vi "AudioTest.Check if Mic and Speaker Operate.vi"() -> ()   [LabVIEW 2018]
uses:
  Functional Test/TypeDefs/FunctTest.Test Item with 2D Image for Instructions, Pass is Indicator Only.ctl
  Functional Test/TypeDefs/FunctTest.Result State.ctl
  Common/Instruments/Audio/Audio Play Record/Audio.Play Signal Setup.ctl
  Common/Instruments/Audio/Audio Play Record/Audio.Record Signal Setup.ctl
  <vilib>/KATE/Queues/Queue Utils.lvlib
panel:
  out "CL Args":string[](array[string])
  out "Output file":path
  out "error out":errorcluster
  out "Running":bool
  in  "Run All Audio Tests":bool
  in  "Run Audio Right Test":bool
  in  "Run Audio Left Test":bool
  in  "Run Audio Mic Test":bool
  out "Test Run Time(s)":dbl format="%.3f"
  out "Left Speaker Spectrum":T1(graph)
  out "Left Test Result":T2
  out "Left Rec Tones (Hz)":dbl[](array[numeric])
  out "Right Rec Tones (Hz)":dbl[](array[numeric])
  out "Right Speaker Spectrum":T1(graph)
  out "Right Test Result":T2
  out "Mic Rec Tones (Hz)":dbl[](array[numeric])
  out "Microphone Spectrum":T1(graph)
  out "Mic Test Result":T2
  in  "Tol%":dbl=3.0 caption="Tone Tolerance(+/-%)"
  in  "RtSetup":T3={"Play Device"="Utah", "Play Volume"=90.0, "DTMF Channel"=7, "Rec Device"="Jabra"} caption="Right Speaker Test Setup"
  in  "LftSetup":T3={"Play Device"="Utah", "Play Volume"=90.0, "DTMF Channel"=4, "Rec Device"="Jabra"} caption="Left Speaker Test Setup"
  in  "MicSetup":T3={"Play Device"="Jabra", "Play Volume"=60.0, "DTMF Channel"=1, "Rec Device"="Valve"} caption="Microphone Test Setup"
  in  "ToneThr":dbl=0.0005 caption="Tone Threshold"
  in  "Sample Rate":dbl=44100.0
  in  "ToneDur":dbl=0.35 caption="Tone Duration(s)"
  out "Audio Test":T4
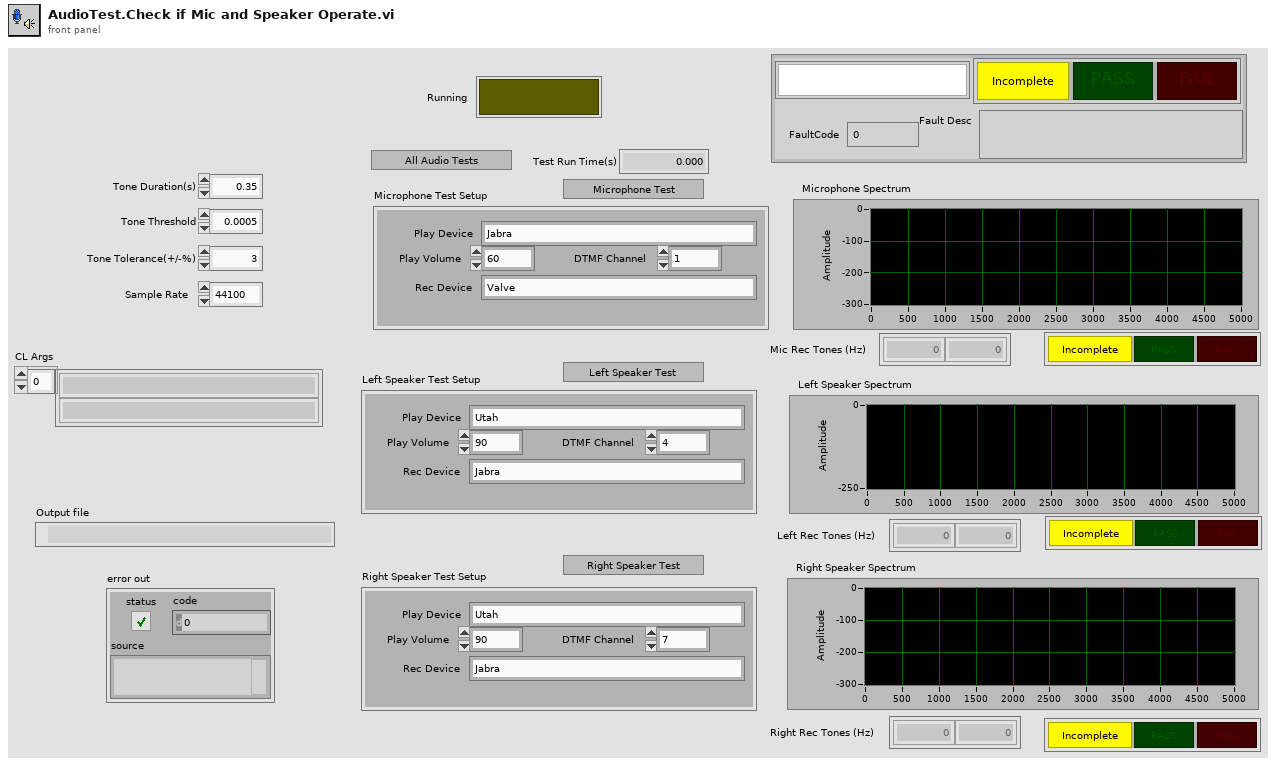
[diagram p1: front panel]
types:
  T1 = cluster{"f0":dbl, "df":dbl, "dB Spectrum (Hann)":dbl[]}
  T2 = typedef "FunctTest.Result State.ctl" = enum32{"NoTest", "PASS", "FAIL"}
  T3 = cluster{"Play Device":string, "Play Volume":dbl, "DTMF Channel":i32, "Rec Device":string}
  T4 = typedef "FunctTest.Test Item with 2D Image for Instructions, Pass is Indicator Only.ctl" = cluster{"Name":picture, "Result":T2, "FaultCode":i32, "Fault Desc":string, "Disabled":bool}
  T5 = enum32{"invalid app kind", "Development System", "Run Time System", "Student Edition", "Embedded LabVIEW", "Evaluation", "Custom"}
  T6 = enum32{"Invalid", "Standard", "Closed", "Hidden", "Minimized", "Maximized"}
  T7 = typedef "Audio.Record Signal Setup.ctl" = cluster{"Device":string, "Left En":bool, "Right En":bool, "PrePlaySec":dbl, "PostPlaySec":dbl}
  T8 = typedef "Audio.Play Signal Setup.ctl" = cluster{"Device":string, "Left En":bool, "Right En":bool, "Volume(%)":dbl, "Amplitude":dbl}
  T9 = cluster{"ToneDur":dbl, "Sample Rate":dbl, "ToneThr":dbl, "Tol%":dbl, "MicSetup":cluster{"Play Device":string, "Play Volume":dbl, "DTMF Channel":i32, "Rec Device":string}, "RtSetup":cluster{"Play Device":string, "Play Volume":dbl, "DTMF Channel":i32, "Rec Device":string}, "LftSetup":cluster{"Play Device":string, "Play Volume":dbl, "DTMF Channel":i32, "Rec Device":string}, "Start":dbl, "CLI":string[], "Out Dir":path, "Faults":errorcluster[]}
  T10 = cluster{"frequency":dbl, "amplitude":dbl, "phase":dbl}[]
  T11 = cluster{"detected frequency":dbl, "detected amplitude":dbl, "detected phase (deg)":dbl}[]
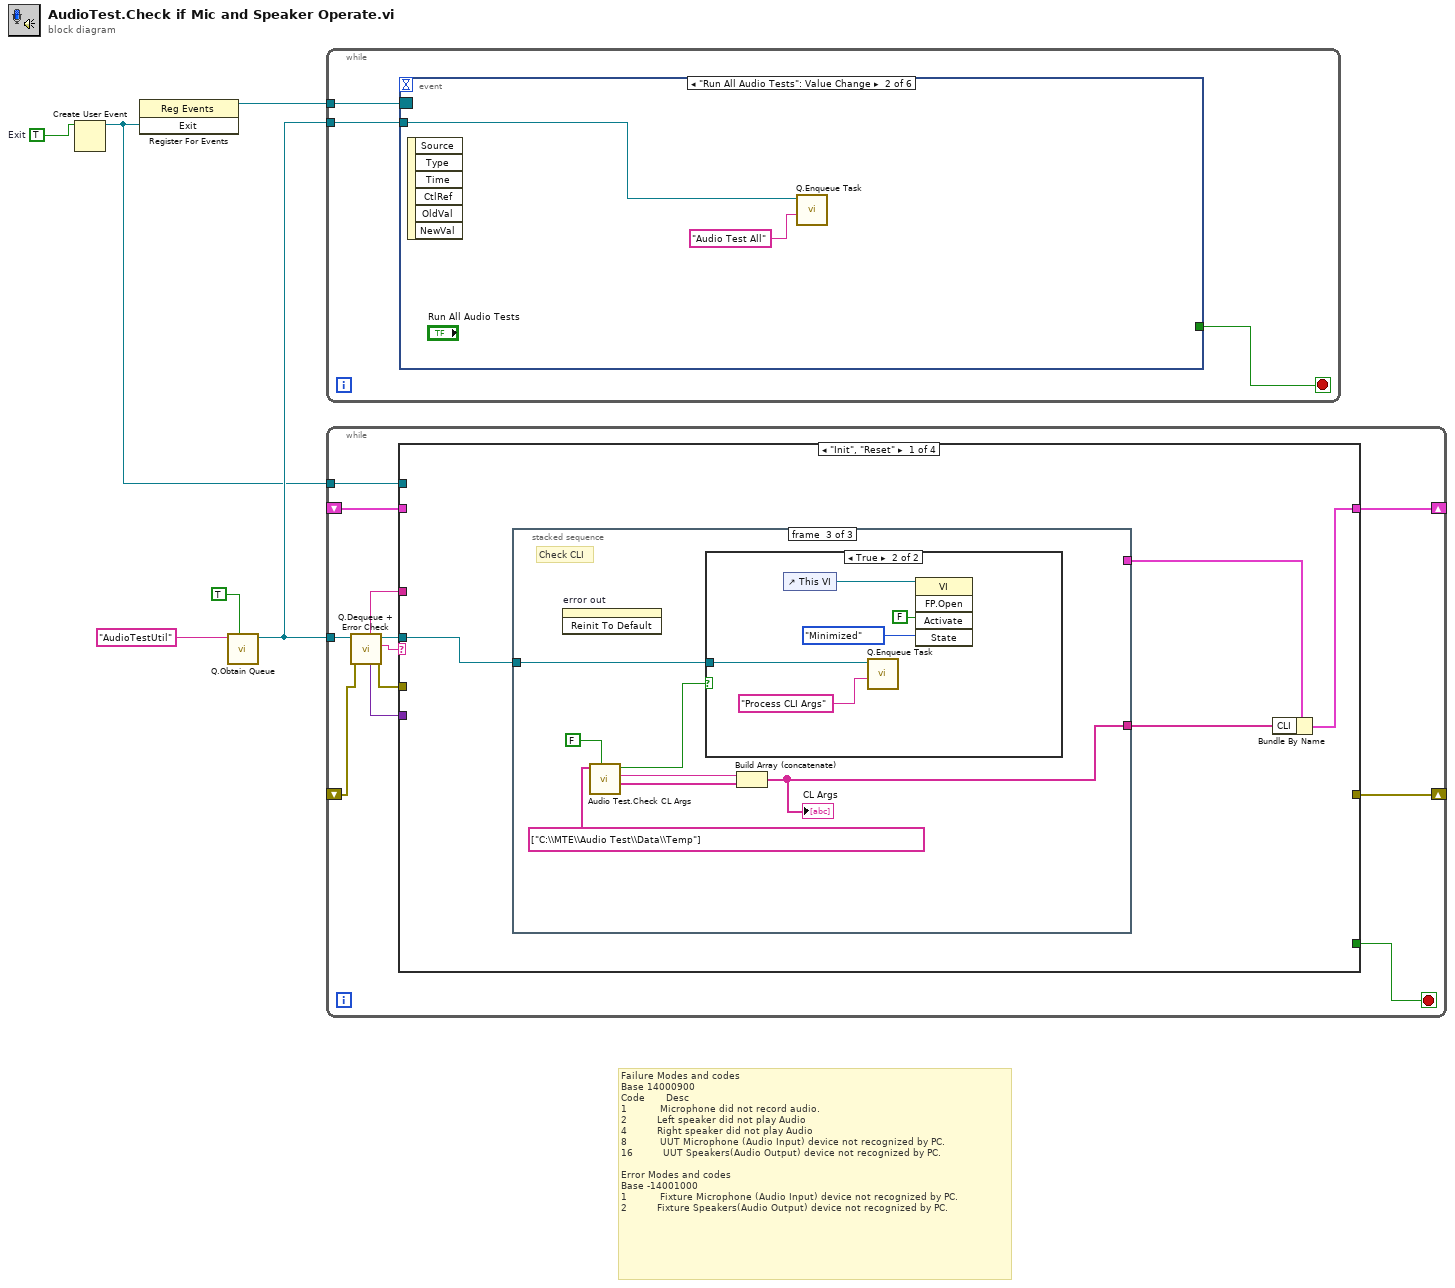
[diagram p0: block diagram]
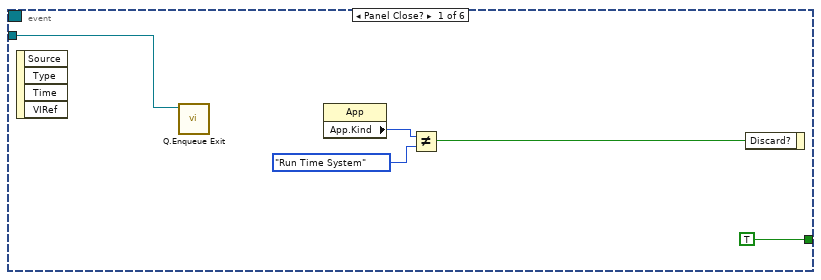
[diagram p2: hidden frame]
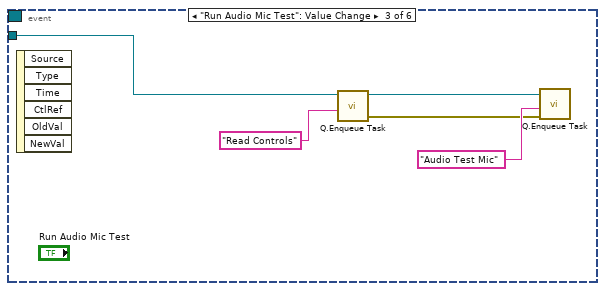
[diagram p3: hidden frame]
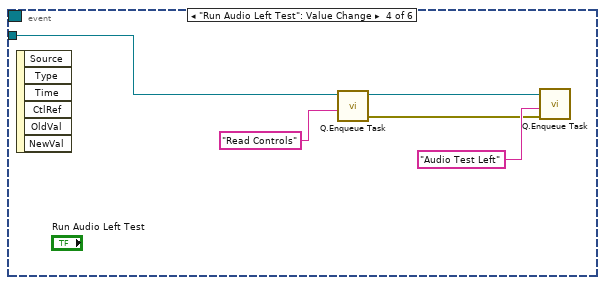
[diagram p4: hidden frame]
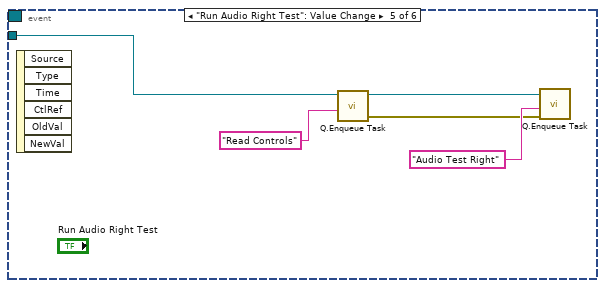
[diagram p5: hidden frame]
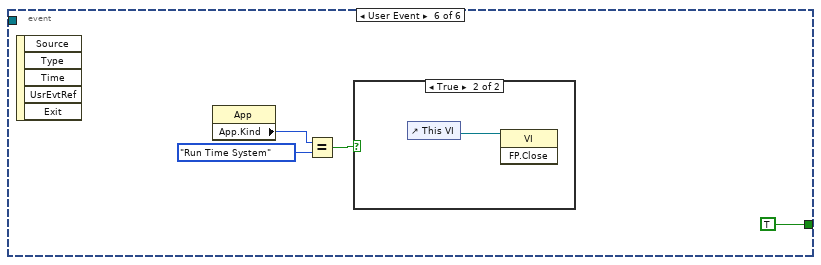
[diagram p6: hidden frame]
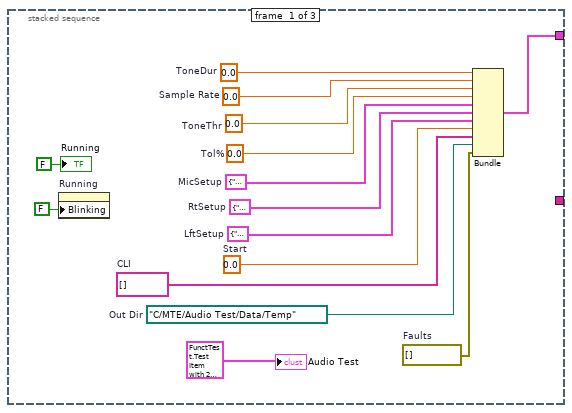
[diagram p8: hidden frame]
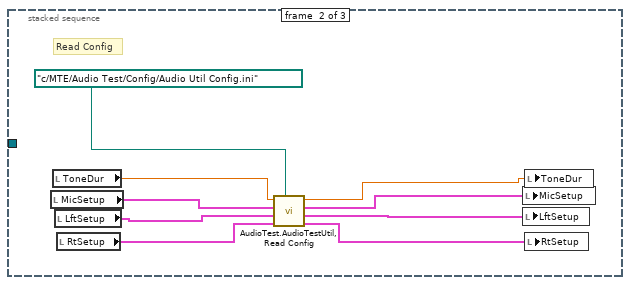
[diagram p9: hidden frame]
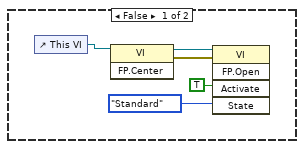
[diagram p10: hidden frame]
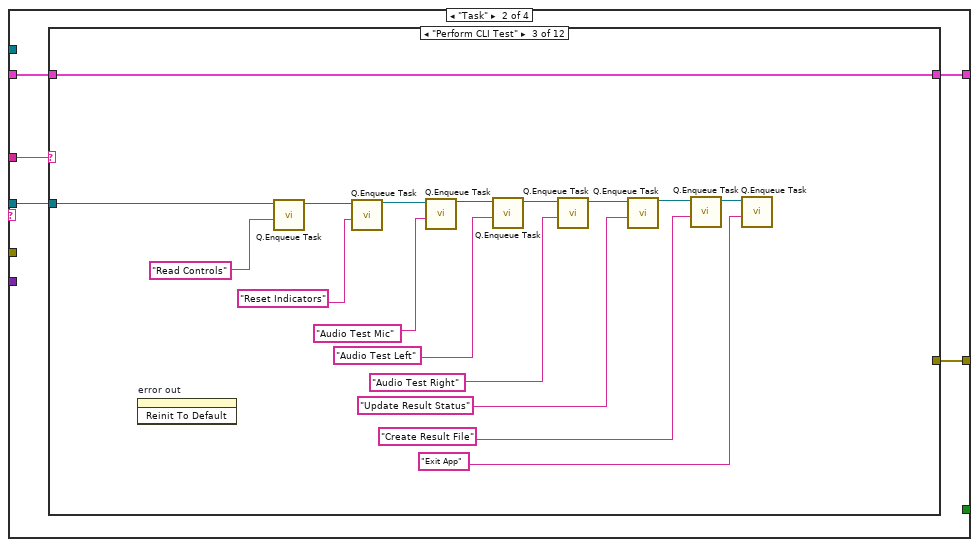
[diagram p11: hidden frame]
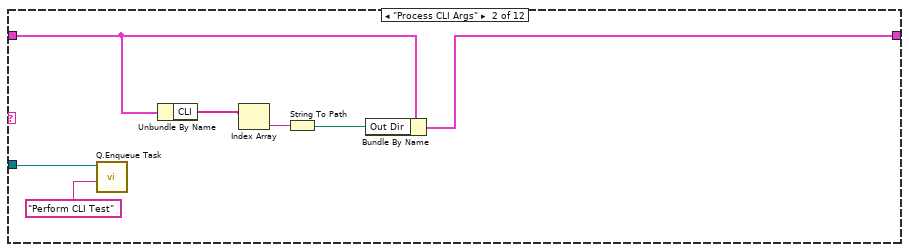
[diagram p13: hidden frame]
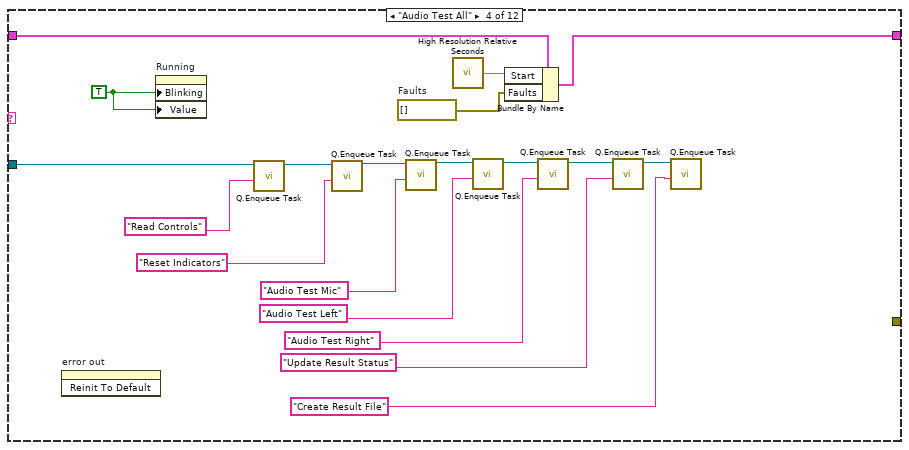
[diagram p14: hidden frame]
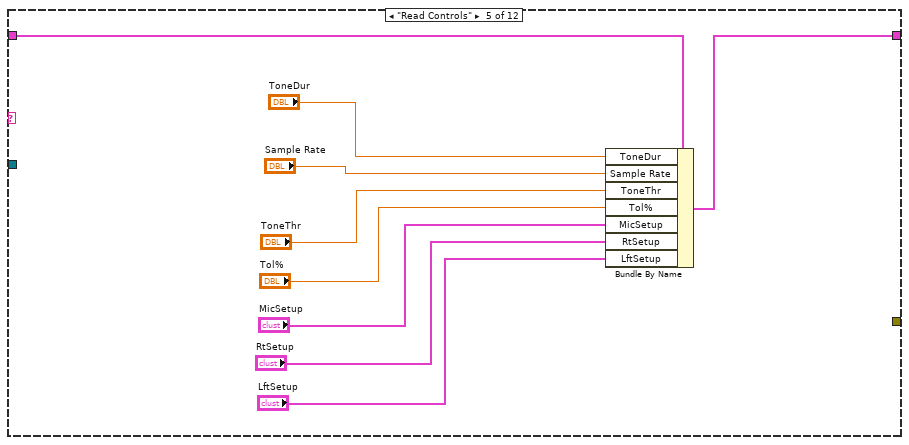
[diagram p15: hidden frame]
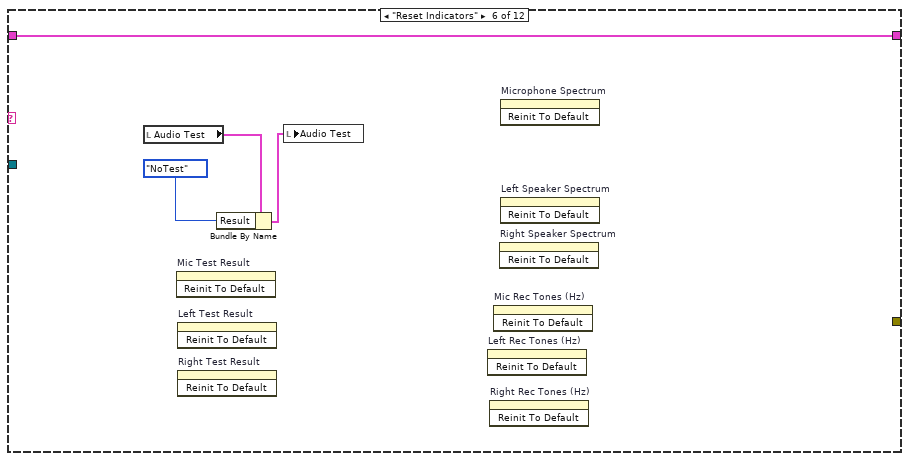
[diagram p16: hidden frame]
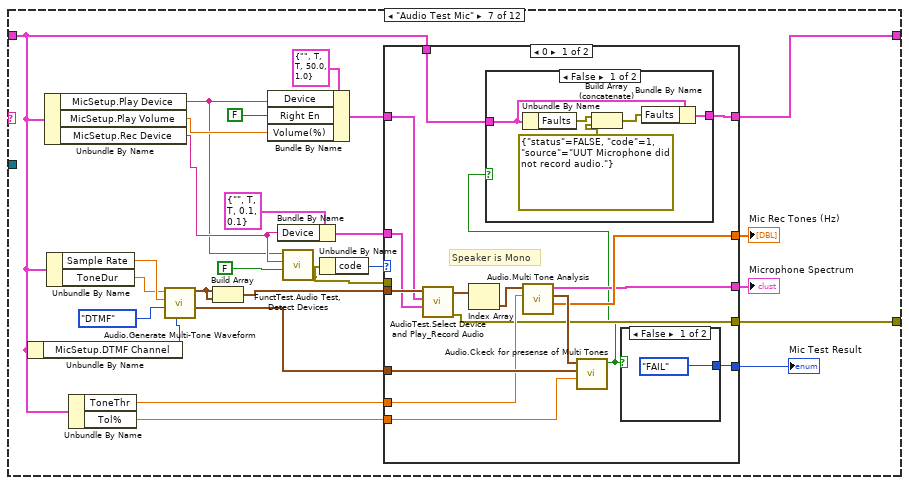
[diagram p17: hidden frame]
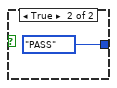
[diagram p19: hidden frame]
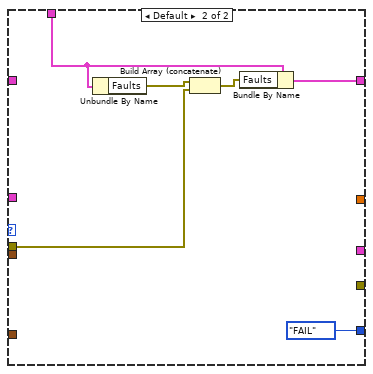
[diagram p20: hidden frame]
diagram:
  w2 = TRUE  # Exit
  # "Failure Modes and codes\nBase 14000900\nCode       Desc\n1           Microphone did not record audio.\n2          Left speaker did not play Audio\n4          Right speaker did not play Audio\n8           UUT Microphone (Audio Input) device not recognized by PC.\n16          UUT Speakers(Audio Output) device not recognized by PC.\n\nError Modes and codes\nBase -14001000\n1           Fixture Microphone (Audio Input) device not recognized by PC.\n2          Fixture Speakers(Audio Output) device not recognized by PC."
  n1 = Create User Event(user event datatype=w2) -> (user event=w1:refnum<user-event>)  [unwired: 1 in, 1 out]
  n2 = register-events(w1) -> (reference out=w3:refnum<event-registration>)  [unwired: 2 in, 1 out]
  n3 = call <vilib>:"Q.Obtain Queue.vi"("Enqueue Init"=TRUE, "Q Name"="AudioTestUtil") -> ("Q Out"=w4:refnum<queue>)  [unwired: 7 in, 2 out]
  n4 = while {
    tunnel: w4 -> [w8]
    tunnel: w3 -> [w7]
    stop <- w9 stop-if-true
    n5 = event shown="[1] \"Run All Audio Tests\": Value Change" {
      selector: w7 -> [_ _ _ _ _ _]
      dyn-events: _ -> [_ _ _ _ _ _]
      timeout: _ -> [_ _ _ _ _ _]
      tunnel: [TRUE _ _ _ _ TRUE] -> w9
      tunnel: w8 -> [w10 w15 w18 w23 w28 _]
      event Panel Close? {
        n6 = event-data() -> ()  [unwired: 1 in, 4 out]
        n7 = call <vilib>:"Q.Enqueue Exit.vi"("Q In"=w10) -> ()  [unwired: 9 in, 2 out]
        n8 = property class="App"() -> ("App.Kind"=w14:T5)  [unwired: 2 in, 2 out]
        n9 = Not Equal?(x=w14, y=T5."Run Time System") -> (x != y?=w12:bool)
        n10 = event-data("Discard?"=w12) -> ()  [unwired: 1 in, 1 out]
      }
      event "Run All Audio Tests": Value Change {
        n11 = event-data() -> ()  [unwired: 1 in, 6 out]
        n12 = call <vilib>:"Q.Enqueue Task.vi"("Task Name"="Audio Test All", "Q In"=w15) -> ()  [unwired: 8 in, 2 out]
      }
      event "Run Audio Mic Test": Value Change {
        n13 = event-data() -> ()  [unwired: 1 in, 6 out]
        n14 = call <vilib>:"Q.Enqueue Task.vi"("Task Name"="Read Controls", "Q In"=w18) -> ("error out"=w19:errorcluster, "Q Out"=w17:refnum<queue>)  [unwired: 8 in]
        n15 = call <vilib>:"Q.Enqueue Task.vi"("Error In"=w19, "Task Name"="Audio Test Mic", "Q In"=w17) -> ()  [unwired: 7 in, 2 out]
      }
      event "Run Audio Left Test": Value Change {
        n16 = event-data() -> ()  [unwired: 1 in, 6 out]
        n17 = call <vilib>:"Q.Enqueue Task.vi"("Task Name"="Read Controls", "Q In"=w23) -> ("error out"=w24:errorcluster, "Q Out"=w22:refnum<queue>)  [unwired: 8 in]
        n18 = call <vilib>:"Q.Enqueue Task.vi"("Error In"=w24, "Task Name"="Audio Test Left", "Q In"=w22) -> ()  [unwired: 7 in, 2 out]
      }
      event "Run Audio Right Test": Value Change {
        n19 = event-data() -> ()  [unwired: 1 in, 6 out]
        n20 = call <vilib>:"Q.Enqueue Task.vi"("Task Name"="Read Controls", "Q In"=w28) -> ("error out"=w29:errorcluster, "Q Out"=w27:refnum<queue>)  [unwired: 8 in]
        n21 = call <vilib>:"Q.Enqueue Task.vi"("Error In"=w29, "Task Name"="Audio Test Right", "Q In"=w27) -> ()  [unwired: 7 in, 2 out]
      }
      event User Event {
        n22 = event-data() -> ()  [unwired: 1 in, 5 out]
        n23 = property class="App"() -> ("App.Kind"=w34:T5)  [unwired: 2 in, 2 out]
        n24 = Equal?(x=w34, y=T5."Run Time System") -> (x = y?=w32:bool)
        n25 = case shown="True" w32 {
          frame False {
          }
          frame True {
            n26 = control-ref of="This VI"() -> (w36:refnum<vi>)
            n27 = invoke class="VI" method="FP.Close"(reference=w36) -> ()  [unwired: 2 in, 3 out]
          }
        }
      }
    }
  }
  n28 = while {
    tunnel: w4 -> [w45]
    shift-right: [w43] -> _
    shift-left: _ -> [w44]
    shift-right: [w41] -> _
    shift-left: _ -> [w40]
    tunnel: w1 -> [w38]
    stop <- w42 stop-if-true
    n29 = call <vilib>:"Q.Dequeue + Error Check.vi"("Error In"=w40, "Q In"=w45) -> ("error out"=w39:errorcluster, "Cmd"=w48:string, "Q Out"=w47:refnum<queue>, "Data1"=w37:variant, "Sub"=w46:string)  [unwired: 4 in, 1 out]
    n30 = case shown="\"Init\", \"Reset\"" w48 {
      tunnel: w47 -> [w52 w94 _ _]
      tunnel: w46 -> [_ w98 w410 _]
      tunnel: w44 -> [_ w97 w411 w419]
      tunnel: [w50 w96 w411 w419] -> w43
      tunnel: [_ _ _ TRUE] -> w42
      tunnel: [_ w95 _ _] -> w41
      tunnel: w39 -> [_ _ w409 _]
      tunnel: w38 -> [_ _ _ w417]
      tunnel: w37 -> [_ _ w408 _]
      frame "Init", "Reset" {
        n31 = stacked-sequence {
          tunnel: [w60 _ _] -> w51
          tunnel: w52 -> [_ _ w83]
          tunnel: [_ _ w78] -> w49
          frame #0 {
            w53 = errorcluster[] []  # Faults
            w54 = path "C:/MTE/Audio Test/Data/Temp"  # Out Dir
            w55 = string[] []  # CLI
            w59 = 0.0  # Start
            w61 = T3 {"Play Device"="", "Play Volume"=0.0, "DTMF Channel"=0, "Rec Device"=""}  # LftSetup
            w62 = T3 {"Play Device"="", "Play Volume"=0.0, "DTMF Channel"=0, "Rec Device"=""}  # RtSetup
            w63 = T3 {"Play Device"="", "Play Volume"=0.0, "DTMF Channel"=0, "Rec Device"=""}  # MicSetup
            w64 = 0.0  # Tol%
            w65 = 0.0  # ToneThr
            w66 = 0.0  # Sample Rate
            w67 = 0.0  # ToneDur
            n32 = property on="Running" class="Bool (strict)"("Blinking"=FALSE) -> ()  [unwired: 2 in, 2 out]
            n33 = Bundle("ToneDur"=w67, "Sample Rate"=w66, "ToneThr"=w65, "Tol%"=w64, "MicSetup"=w63, "RtSetup"=w62, "LftSetup"=w61, "Start"=w59, "CLI"=w55, "Out Dir"=w54, "Faults"=w53) -> (w60:T9)  [unwired: 1 in]
            "Running" <- FALSE ("Running")
            "Audio Test" <- T4 {"Name"=bytes[74], "Result"=enum."NoTest", "FaultCode"=0, "Fault Desc"="", "Disabled"=TRUE} ("Audio Test")
          }
          frame #1 {
            # "Read Config"
            n34 = local read "MicSetup"() -> (w74:T3)
            n35 = local read "ToneDur"() -> (w76:dbl)
            n36 = local read "LftSetup"() -> (w73:T3)
            n37 = local read "RtSetup"() -> (w72:T3)
            n38 = call "AudioTest.AudioTestUtil, Read Config.vi"("File"=path "c:/MTE/Audio Test/Config/Audio Util Config.ini", "RtSetup"=w72, "LftSetup"=w73, "MicSetup"=w74, "ToneDur"=w76) -> ("RtSetup Out"=w68:T3, "LftSetup Out"=w69:T3, "MicSetup Out"=w70:T3, "ToneDur Out"=w71:dbl)  [unwired: 2 in, 1 out]
            n39 = local write "MicSetup"(w70) -> ()
            n40 = local write "LftSetup"(w69) -> ()
            n41 = local write "ToneDur"(w71) -> ()
            n42 = local write "RtSetup"(w68) -> ()
          }
          frame #2 {
            # "Check CLI"
            n43 = invoke on="error out" class="Clust (strict)" method="Reinit To Default"() -> ()  [unwired: 3 in, 3 out]
            n44 = call "Audio Test.Check CL Args.vi"("Simulate"=FALSE, "Sim CL Args"=string[] ["C:\\MTE\\Audio Test\\Data\\Temp"]) -> ("Args"=w77:string[], "Action"=w81:string, "CmdLine"=w82:bool)  [unwired: 7 in]
            n45 = case shown="True" w82 {
              tunnel: w83 -> [_ w92]
              frame False {
                n46 = control-ref of="This VI"() -> (w86:refnum<vi>)
                n47 = invoke class="VI" method="FP.Center"(reference=w86) -> (reference out=w87:refnum<vi>, error out=w88:errorcluster)  [unwired: 2 in, 1 out]
                n48 = invoke class="VI" method="FP.Open"(reference=w87, error in=w88, "Activate"=TRUE ("Activate?"), "State"=T6."Standard") -> ()  [unwired: 1 in, 5 out]
              }
              frame True {
                n49 = control-ref of="This VI"() -> (w89:refnum<vi>)
                n50 = call <vilib>:"Q.Enqueue Task.vi"("Task Name"="Process CLI Args", "Q In"=w92) -> ()  [unwired: 8 in, 2 out]
                n51 = invoke class="VI" method="FP.Open"(reference=w89, "Activate"=FALSE ("Activate?"), "State"=T6."Minimized") -> ()  [unwired: 2 in, 5 out]
              }
            }
            n52 = Build Array (concatenate)(w81, w77) -> (w78:string[])
            "CL Args" <- w78
          }
        }
        n53 = Bundle By Name(cluster=w51, "CLI"=w49) -> (w50:T9)
      }
      frame "Task" {
        n54 = case shown="\"Perform CLI Test\"" w98 {
          tunnel: w97 -> [w99 w100 w123 w128 w143 w155 w156 w215 w271 w338 w404 w406]
          tunnel: [w99 w101 w123 w129 w144 w155 w157 w213 w268 w338 w404 w406] -> w96
          tunnel: [_ _ _ _ _ _ w172 w228 w283 _ w389 _] -> w95
          tunnel: w94 -> [_ w105 w111 w131 _ _ _ _ _ _ _ w405]
          frame Default {
          }
          frame "Process CLI Args" {
            n55 = call <vilib>:"Q.Enqueue Task.vi"("Task Name"="Perform CLI Test", "Q In"=w105) -> ()  [unwired: 8 in, 2 out]
            n56 = Unbundle By Name(w100) -> ("CLI"=w104:string[])
            n57 = Index Array(array=w104) -> (element=w103:string)  [unwired: 1 in]
            n58 = String To Path(string=w103) -> (path=w102:path)
            n59 = Bundle By Name(cluster=w100, "Out Dir"=w102) -> (w101:T9)
          }
          frame "Perform CLI Test" {
            n60 = invoke on="error out" class="Clust (strict)" method="Reinit To Default"() -> ()  [unwired: 3 in, 3 out]
            n61 = call <vilib>:"Q.Enqueue Task.vi"("Task Name"="Read Controls", "Q In"=w111) -> ("Q Out"=w113:refnum<queue>)  [unwired: 8 in, 1 out]
            n62 = call <vilib>:"Q.Enqueue Task.vi"("Task Name"="Reset Indicators", "Q In"=w113) -> ("Q Out"=w117:refnum<queue>)  [unwired: 8 in, 1 out]
            n63 = call <vilib>:"Q.Enqueue Task.vi"("Task Name"="Audio Test Mic", "Q In"=w117) -> ("Q Out"=w122:refnum<queue>)  [unwired: 8 in, 1 out]
            n64 = call <vilib>:"Q.Enqueue Task.vi"("Task Name"="Audio Test Left", "Q In"=w122) -> ("Q Out"=w121:refnum<queue>)  [unwired: 8 in, 1 out]
            n65 = call <vilib>:"Q.Enqueue Task.vi"("Task Name"="Audio Test Right", "Q In"=w121) -> ("Q Out"=w115:refnum<queue>)  [unwired: 8 in, 1 out]
            n66 = call <vilib>:"Q.Enqueue Task.vi"("Task Name"="Update Result Status", "Q In"=w115) -> ("Q Out"=w110:refnum<queue>)  [unwired: 8 in, 1 out]
            n67 = call <vilib>:"Q.Enqueue Task.vi"("Task Name"="Create Result File", "Q In"=w110) -> ("Q Out"=w108:refnum<queue>)  [unwired: 8 in, 1 out]
            n68 = call <vilib>:"Q.Enqueue Task.vi"("Task Name"="Exit App", "Q In"=w108) -> ()  [unwired: 8 in, 2 out]
          }
          frame "Audio Test All" {
            w124 = errorcluster[] []  # Faults
            w133 = TRUE ("Blinking")
            n69 = invoke on="error out" class="Clust (strict)" method="Reinit To Default"() -> ()  [unwired: 3 in, 3 out]
            n70 = property on="Running" class="Bool (strict)"("Blinking"=w133, "Value"=w133) -> ()  [unwired: 2 in, 2 out]
            n71 = call <vilib>:"Q.Enqueue Task.vi"("Task Name"="Read Controls", "Q In"=w131) -> ("Q Out"=w132:refnum<queue>)  [unwired: 8 in, 1 out]
            n72 = call <vilib>:"Q.Enqueue Task.vi"("Task Name"="Reset Indicators", "Q In"=w132) -> ("Q Out"=w137:refnum<queue>)  [unwired: 8 in, 1 out]
            n73 = call <vilib>:"Q.Enqueue Task.vi"("Task Name"="Audio Test Mic", "Q In"=w137) -> ("Q Out"=w142:refnum<queue>)  [unwired: 8 in, 1 out]
            n74 = call <vilib>:"High Resolution Relative Seconds.vi"() -> ("relative seconds"=w127:dbl)
            n75 = call <vilib>:"Q.Enqueue Task.vi"("Task Name"="Audio Test Left", "Q In"=w142) -> ("Q Out"=w141:refnum<queue>)  [unwired: 8 in, 1 out]
            n76 = Bundle By Name(cluster=w128, "Start"=w127, "Faults"=w124) -> (w129:T9)
            n77 = call <vilib>:"Q.Enqueue Task.vi"("Task Name"="Audio Test Right", "Q In"=w141) -> ("Q Out"=w135:refnum<queue>)  [unwired: 8 in, 1 out]
            n78 = call <vilib>:"Q.Enqueue Task.vi"("Task Name"="Update Result Status", "Q In"=w135) -> ("Q Out"=w125:refnum<queue>)  [unwired: 8 in, 1 out]
            n79 = call <vilib>:"Q.Enqueue Task.vi"("Task Name"="Create Result File", "Q In"=w125) -> ()  [unwired: 8 in, 2 out]
          }
          frame "Read Controls" {
            n80 = Bundle By Name(cluster=w143, "ToneDur"="ToneDur", "Sample Rate"="Sample Rate", "ToneThr"="ToneThr", "Tol%"="Tol%", "MicSetup"="MicSetup", "RtSetup"="RtSetup", "LftSetup"="LftSetup") -> (w144:T9)
          }
          frame "Reset Indicators" {
            n81 = local read "Audio Test"() -> (w154:T4)
            n82 = invoke on="Mic Test Result" class="RadioBtnsControl (strict)" method="Reinit To Default"() -> ()  [unwired: 3 in, 3 out]
            n83 = invoke on="Left Test Result" class="RadioBtnsControl (strict)" method="Reinit To Default"() -> ()  [unwired: 3 in, 3 out]
            n84 = invoke on="Right Test Result" class="RadioBtnsControl (strict)" method="Reinit To Default"() -> ()  [unwired: 3 in, 3 out]
            n85 = Bundle By Name(cluster=w154, "Result"=FunctTest.Result_State."NoTest") -> (w153:T4)
            n86 = local write "Audio Test"(w153) -> ()
            n87 = invoke on="Left Rec Tones (Hz)" class="Arr (strict)" method="Reinit To Default"() -> ()  [unwired: 3 in, 3 out]
            n88 = invoke on="Right Rec Tones (Hz)" class="Arr (strict)" method="Reinit To Default"() -> ()  [unwired: 3 in, 3 out]
            n89 = invoke on="Mic Rec Tones (Hz)" class="Arr (strict)" method="Reinit To Default"() -> ()  [unwired: 3 in, 3 out]
            n90 = invoke on="Right Speaker Spectrum" class="WFGraph (strict)" method="Reinit To Default"() -> ()  [unwired: 3 in, 3 out]
            n91 = invoke on="Microphone Spectrum" class="WFGraph (strict)" method="Reinit To Default"() -> ()  [unwired: 3 in, 3 out]
            n92 = invoke on="Left Speaker Spectrum" class="WFGraph (strict)" method="Reinit To Default"() -> ()  [unwired: 3 in, 3 out]
          }
          frame "Audio Test Mic" {
            n93 = Unbundle By Name(w156) -> ("MicSetup.DTMF Channel"=w171:i32)
            n94 = Unbundle By Name(w156) -> ("MicSetup.Play Device"=w161:string, "MicSetup.Play Volume"=w169:dbl, "MicSetup.Rec Device"=w162:string)
            n95 = Unbundle By Name(w156) -> ("Sample Rate"=w177:dbl, "ToneDur"=w163:dbl)
            n96 = Unbundle By Name(w156) -> ("ToneThr"=w176:dbl, "Tol%"=w175:dbl)
            n97 = call "Audio.Generate Multi-Tone Waveform.vi"("DTMF Num"=w171, "Type"=enum16{"User Specified", "DTMF"}."DTMF", "Sample Rate"=w177, "Dur(s)"=w163) -> ("Tones Out"=w178:T10, "Waveform"=w180:waveform(dbl))  [unwired: 6 in]
            n98 = Build Array(w180, w180) -> (w179:waveform(dbl)[])
            n99 = Bundle By Name(cluster=T8 {"Device"="", "Left En"=TRUE, "Right En"=TRUE, "Volume(%)"=50.0, "Amplitude"=1.0} ("Play Setup"), "Device"=w161, "Right En"=FALSE, "Volume(%)"=w169) -> (w170:T8)
            n100 = Bundle By Name(cluster=T7 {"Device"="", "Left En"=TRUE, "Right En"=TRUE, "PrePlaySec"=0.1, "PostPlaySec"=0.1} ("Rec Setup"), "Device"=w162) -> (w167:T7)
            n101 = call "FunctTest.Audio Test, Detect Devices.vi"("UUT is Mic(F)\\Speaker(T)"=FALSE ("UUT is Mic(F)\\Speaker(T)"), "Mic Device"=w162, "Speaker Device"=w161) -> ("error out"=w158:errorcluster)  [unwired: 8 in]
            n102 = Unbundle By Name(w158) -> ("code"=w159:i32)
            n103 = case shown="0" w159 {
              tunnel: w179 -> [w197 _]
              tunnel: w178 -> [w193 _]
              tunnel: w176 -> [w192 _]
              tunnel: w175 -> [w191 _]
              tunnel: [w190 _] -> w172
              tunnel: w170 -> [w189 _]
              tunnel: w167 -> [w188 _]
              tunnel: [w187 _] -> w166
              tunnel: [w186 _] -> w165
              tunnel: [w185 FunctTest.Result_State."FAIL" ("Left Test Result")] -> w164
              tunnel: w158 -> [_ w208]
              tunnel: w156 -> [w183 w210]
              tunnel: [w184 w206] -> w157
              frame 0 {
                # "Speaker is Mono"
                n104 = call "AudioTest.Select Device and Play_Record Audio.vi"("Rec Setup"=w188, "Play Setup"=w189, "Play Wvfrm"=w197) -> ("error out"=w190:errorcluster, "Rec Wvfrm"=w196:waveform(dbl)[])  [unwired: 7 in]
                n105 = Index Array(array=w196) -> (element=w195:waveform(dbl))  [unwired: 1 in]
                n106 = call "Audio.Multi Tone Analysis.vi"("threshold"=w192, "Wvfrm In"=w195) -> ("Tones"=w187:dbl[], "multiple tone information"=w194:T11, "Spectrum"=w186:T1)  [unwired: 7 in]
                n107 = call "Audio.Ckeck for presense of Multi Tones.vi"("Tolerance(+/-%)"=w191, "Stimulus Tones"=w193, "Detected Tones"=w194) -> ("Pass"=w182:bool)  [unwired: 8 in]
                n108 = case shown="False" w182 {
                  tunnel: [w200 w203] -> w184
                  tunnel: w183 -> [w199 w203]
                  frame False {
                    n109 = Unbundle By Name(w199) -> ("Faults"=w201:errorcluster[])
                    n110 = Build Array (concatenate)(w201, errorcluster {"status"=FALSE, "code"=1, "source"="UUT Microphone did not record audio."} ("error constant")) -> (w202:errorcluster[])
                    n111 = Bundle By Name(cluster=w199, "Faults"=w202) -> (w200:T9)
                  }
                  frame True {
                  }
                }
                n112 = case shown="False" w182 {
                  tunnel: [FunctTest.Result_State."FAIL" ("Left Test Result") FunctTest.Result_State."PASS" ("Left Test Result")] -> w185
                  frame False {
                  }
                  frame True {
                  }
                }
              }
              frame Default {
                n113 = Unbundle By Name(w210) -> ("Faults"=w209:errorcluster[])
                n114 = Build Array (concatenate)(w209, w208) -> (w211:errorcluster[])
                n115 = Bundle By Name(cluster=w210, "Faults"=w211) -> (w206:T9)
              }
            }
            "Mic Rec Tones (Hz)" <- w166
            "Microphone Spectrum" <- w165
            "Mic Test Result" <- w164
          }
          frame "Audio Test Right" {
            n116 = Unbundle By Name(w215) -> ("RtSetup.DTMF Channel"=w227:i32)
            n117 = Unbundle By Name(w215) -> ("Sample Rate"=w233:dbl, "ToneDur"=w219:dbl)
            n118 = Unbundle By Name(w215) -> ("RtSetup.Play Device"=w217:string, "RtSetup.Play Volume"=w225:dbl, "RtSetup.Rec Device"=w216:string)
            n119 = Unbundle By Name(w215) -> ("ToneThr"=w232:dbl, "Tol%"=w231:dbl)
            n120 = call "Audio.Generate Multi-Tone Waveform.vi"("DTMF Num"=w227, "Type"=enum16{"User Specified", "DTMF"}."DTMF", "Sample Rate"=w233, "Dur(s)"=w219) -> ("Tones Out"=w234:T10, "Waveform"=w236:waveform(dbl))  [unwired: 6 in]
            n121 = Build Array(w236, w236) -> (w235:waveform(dbl)[])
            n122 = call "AudioTest.Audio Test, Detect Devices.vi"("UUT is Mic(F)\\Speaker(T)"=TRUE ("UUT is Mic(F)\\Speaker(T)"), "Mic Device"=w216, "Speaker Device"=w217) -> ("error out"=w212:errorcluster)  [unwired: 8 in]
            n123 = Bundle By Name(cluster=T8 {"Device"="", "Left En"=TRUE, "Right En"=TRUE, "Volume(%)"=50.0, "Amplitude"=1.0} ("Play Setup"), "Device"=w217, "Left En"=FALSE ("Right En"), "Volume(%)"=w225) -> (w226:T8)
            n124 = Bundle By Name(cluster=T7 {"Device"="", "Left En"=TRUE, "Right En"=TRUE, "PrePlaySec"=0.1, "PostPlaySec"=0.1} ("Rec Setup"), "Device"=w216) -> (w223:T7)
            n125 = Unbundle By Name(w212) -> ("code"=w214:i32)
            n126 = case shown="0" w214 {
              tunnel: w235 -> [_ w259]
              tunnel: w234 -> [_ w255]
              tunnel: w232 -> [_ w254]
              tunnel: w231 -> [_ w253]
              tunnel: [_ w252] -> w228
              tunnel: w226 -> [_ w251]
              tunnel: w223 -> [_ w250]
              tunnel: [FunctTest.Result_State."FAIL" ("Left Test Result") w249] -> w222
              tunnel: [_ w248] -> w221
              tunnel: [_ w247] -> w220
              tunnel: w215 -> [w241 w245]
              tunnel: [w240 w246] -> w213
              tunnel: w212 -> [w239 _]
              frame Default {
                n127 = Unbundle By Name(w241) -> ("Faults"=w242:errorcluster[])
                n128 = Build Array (concatenate)(w242, w239) -> (w243:errorcluster[])
                n129 = Bundle By Name(cluster=w241, "Faults"=w243) -> (w240:T9)
              }
              frame 0 {
                # "Speaker is Mono"
                n130 = call "AudioTest.Select Device and Play_Record Audio.vi"("Rec Setup"=w250, "Play Setup"=w251, "Play Wvfrm"=w259) -> ("error out"=w252:errorcluster, "Rec Wvfrm"=w258:waveform(dbl)[])  [unwired: 7 in]
                n131 = Index Array(array=w258) -> (element=w257:waveform(dbl))  [unwired: 1 in]
                n132 = call "Audio.Multi Tone Analysis.vi"("threshold"=w254, "Wvfrm In"=w257) -> ("Tones"=w247:dbl[], "multiple tone information"=w256:T11, "Spectrum"=w248:T1)  [unwired: 7 in]
                n133 = call "Audio.Ckeck for presense of Multi Tones.vi"("Tolerance(+/-%)"=w253, "Stimulus Tones"=w255, "Detected Tones"=w256) -> ("Pass"=w244:bool)  [unwired: 8 in]
                n134 = case shown="False" w244 {
                  tunnel: [w262 w265] -> w246
                  tunnel: w245 -> [w261 w265]
                  frame False {
                    n135 = Unbundle By Name(w261) -> ("Faults"=w263:errorcluster[])
                    n136 = Build Array (concatenate)(w263, errorcluster {"status"=FALSE, "code"=4, "source"="UUT Right Speaker did not play audio."} ("error constant")) -> (w264:errorcluster[])
                    n137 = Bundle By Name(cluster=w261, "Faults"=w264) -> (w262:T9)
                  }
                  frame True {
                  }
                }
                n138 = case shown="False" w244 {
                  tunnel: [FunctTest.Result_State."FAIL" ("Left Test Result") FunctTest.Result_State."PASS" ("Left Test Result")] -> w249
                  frame False {
                  }
                  frame True {
                  }
                }
              }
            }
            "Right Rec Tones (Hz)" <- w220
            "Right Speaker Spectrum" <- w221
            "Right Test Result" <- w222
          }
          frame "Audio Test Left" {
            w275 = 0.0 ("PrePlaySec")
            n139 = Unbundle By Name(w271) -> ("LftSetup.DTMF Channel"=w282:i32)
            n140 = Unbundle By Name(w271) -> ("Sample Rate"=w288:dbl, "ToneDur"=w276:dbl)
            n141 = Unbundle By Name(w271) -> ("LftSetup.Play Device"=w273:string, "LftSetup.Play Volume"=w280:dbl, "LftSetup.Rec Device"=w272:string)
            n142 = Unbundle By Name(w271) -> ("ToneThr"=w287:dbl, "Tol%"=w286:dbl)
            n143 = call "Audio.Generate Multi-Tone Waveform.vi"("DTMF Num"=w282, "Type"=enum16{"User Specified", "DTMF"}."DTMF", "Sample Rate"=w288, "Dur(s)"=w276) -> ("Tones Out"=w290:T10, "Waveform"=w293:waveform(dbl))  [unwired: 6 in]
            n144 = Build Array(w293, w293) -> (w292:waveform(dbl)[])
            n145 = Bundle By Name(cluster=T7 {"Device"="", "Left En"=TRUE, "Right En"=TRUE, "PrePlaySec"=0.1, "PostPlaySec"=0.1} ("Rec Setup"), "Device"=w272, "PrePlaySec"=w275, "PostPlaySec"=w275) -> (w278:T7)
            n146 = Bundle By Name(cluster=T8 {"Device"="", "Left En"=TRUE, "Right En"=TRUE, "Volume(%)"=50.0, "Amplitude"=1.0} ("Play Setup"), "Device"=w273, "Right En"=FALSE, "Volume(%)"=w280) -> (w281:T8)
            n147 = call "AudioTest.Audio Test, Detect Devices.vi"("UUT is Mic(F)\\Speaker(T)"=TRUE ("UUT is Mic(F)\\Speaker(T)"), "Mic Device"=w272, "Speaker Device"=w273) -> ("error out"=w270:errorcluster)  [unwired: 8 in]
            n148 = Unbundle By Name(w270) -> ("code"=w269:i32)
            n149 = case shown="0" w269 {
              tunnel: w292 -> [_ w316]
              tunnel: [_ w313] -> w291
              tunnel: w290 -> [_ w311]
              tunnel: [FunctTest.Result_State."FAIL" ("Left Test Result") w310] -> w289
              tunnel: w287 -> [_ w309]
              tunnel: w286 -> [_ w308]
              tunnel: [_ w307] -> w283
              tunnel: w281 -> [_ w306]
              tunnel: w278 -> [_ w305]
              tunnel: [_ w304] -> w277
              tunnel: w271 -> [w296 w303]
              tunnel: w270 -> [w295 _]
              tunnel: [w297 w302] -> w268
              frame Default {
                n150 = Unbundle By Name(w296) -> ("Faults"=w298:errorcluster[])
                n151 = Build Array (concatenate)(w298, w295) -> (w299:errorcluster[])
                n152 = Bundle By Name(cluster=w296, "Faults"=w299) -> (w297:T9)
              }
              frame 0 {
                # "Speaker is Mono"
                n153 = call "AudioTest.Select Device and Play_Record Audio.vi"("Rec Setup"=w305, "Play Setup"=w306, "Play Wvfrm"=w316) -> ("error out"=w307:errorcluster, "Rec Wvfrm"=w315:waveform(dbl)[])  [unwired: 7 in]
                n154 = Index Array(array=w315) -> (element=w314:waveform(dbl))  [unwired: 1 in]
                n155 = call "Audio.Multi Tone Analysis.vi"("threshold"=w309, "Wvfrm In"=w314) -> ("Tones"=w304:dbl[], "multiple tone information"=w312:T11, "Spectrum"=w313:T1)  [unwired: 7 in]
                n156 = call "Audio.Ckeck for presense of Multi Tones.vi"("Tolerance(+/-%)"=w308, "Stimulus Tones"=w311, "Detected Tones"=w312) -> ("Pass"=w301:bool)  [unwired: 8 in]
                n157 = case shown="False" w301 {
                  tunnel: [w319 w322] -> w302
                  tunnel: w303 -> [w318 w322]
                  frame False {
                    n158 = Unbundle By Name(w318) -> ("Faults"=w320:errorcluster[])
                    n159 = Build Array (concatenate)(w320, errorcluster {"status"=FALSE, "code"=2, "source"="UUT Left Speaker did not play audio."} ("error constant")) -> (w321:errorcluster[])
                    n160 = Bundle By Name(cluster=w318, "Faults"=w321) -> (w319:T9)
                  }
                  frame True {
                  }
                }
                n161 = case shown="False" w301 {
                  tunnel: [FunctTest.Result_State."FAIL" ("Left Test Result") FunctTest.Result_State."PASS" ("Left Test Result")] -> w310
                  frame False {
                  }
                  frame True {
                  }
                }
              }
            }
            "Left Speaker Spectrum" <- w291
            "Left Test Result" <- w289
            "Left Rec Tones (Hz)" <- w277
          }
          frame "Update Result Status" {
            w344 = FALSE ("Blinking")
            # "Fail"
            # "Error"
            n162 = Unbundle By Name(w338) -> ("Faults"=w326:errorcluster[])
            n163 = call "Error.Remove Duplicate Errors.vi"("Errors In"=w326) -> ("Errors Out"=w325:errorcluster[])  [unwired: 10 in]
            n164 = property on="Running" class="Bool (strict)"("Blinking"=w344, "Value"=w344) -> ()  [unwired: 2 in, 2 out]
            n165 = for {
              tunnel: w325 -> [w369] mode=indexing
              shift-right: [w363] -> w333
              shift-left: 0 -> [w364]
              shift-right: [w361] -> w332
              shift-left: "" -> [w362]
              shift-right: [w366] -> w331
              shift-left: 0 -> [w365]
              shift-right: [w368] -> w330
              shift-left: "" -> [w367]
              n166 = case shown="Error" w369 {
                selector: w369 -> [w378 w388]
                tunnel: [w377 w380] -> w368
                tunnel: w367 -> [w376 w380]
                tunnel: [w374 w381] -> w366
                tunnel: w365 -> [w373 w381]
                tunnel: w364 -> [w371 w383]
                tunnel: [w371 w384] -> w363
                tunnel: w362 -> [w370 w382]
                tunnel: [w370 w385] -> w361
                frame No Error {
                  n167 = Unbundle By Name(w378) -> ("code"=w372:i32, "source"=w375:string)
                  n168 = Add(x=w372, y=w373) -> (x+y=w374:i32)
                  n169 = call "String.Build Delimited List.vi"("New Data"=w375, "Existing Str"=w376) -> ("New Str"=w377:string)  [unwired: 9 in]
                }
                frame Error {
                  n170 = Unbundle By Name(w388) -> ("code"=w386:i32, "source"=w387:string)
                  n171 = Add(x=w386, y=w383) -> (x+y=w384:i32)
                  n172 = call "String.Build Delimited List.vi"("Delimiter"=" ", "New Data"=w387, "Existing Str"=w382) -> ("New Str"=w385:string)  [unwired: 8 in]
                }
              }
            }
            n173 = Unbundle By Name(w338) -> ("Start"=w340:dbl)
            n174 = call <vilib>:"High Resolution Relative Seconds.vi"() -> ("relative seconds"=w341:dbl)
            n175 = Subtract(x=w341, y=w340) -> (x-y=→"Test Run Time(s)":dbl)
            n176 = case shown="0" w333 {
              selector: w333 -> [_ w358]
              tunnel: w332 -> [_ w359]
              tunnel: w331 -> [w349 _]
              tunnel: w330 -> [w347 _]
              tunnel: [w348 FunctTest.Result_State."FAIL" ("Result")] -> w329
              tunnel: [w346 w359] -> w328
              tunnel: [w345 w356] -> w327
              frame 0 {
                n177 = case shown="Default" w349 {
                  selector: w349 -> [w351 _]
                  tunnel: [FunctTest.Result_State."FAIL" ("Result") FunctTest.Result_State."PASS" ("Result")] -> w348
                  tunnel: w347 -> [w353 _]
                  tunnel: [w353 _] -> w346
                  tunnel: [w350 _] -> w345
                  frame Default {
                    n178 = Add(x=14000900, y=w351) -> (x+y=w350:i32)
                  }
                  frame 0 {
                  }
                }
              }
              frame Default {
                # "Error"
                n179 = Subtract(x=-14001000, y=w358) -> (x-y=w356:i32)
              }
            }
            n180 = local read "Audio Test"() -> (w343:T4)
            n181 = Bundle By Name(cluster=w343, "Result"=w329, "Fault Desc"=w328, "FaultCode"=w327) -> (w342:T4)
            n182 = local write "Audio Test"(w342) -> ()
          }
          frame "Create Result File" {
            w397 = "\t"
            n183 = local read "Audio Test"() -> (w401:T4)
            n184 = Unbundle By Name(w401) -> ("Result"=w400:T2, "FaultCode"=w399:i32, "Fault Desc"=w394:string)
            n185 = Format Into String(w400) -> (resulting string=w396:string)  [unwired: 3 in, 1 out]
            n186 = Unbundle By Name(w404) -> ("Out Dir"=w403:path)
            n187 = Number To Decimal String(number=w399) -> (decimal integer string=w395:string)  [unwired: 1 in]
            n188 = Build Path(base path=w403, name or relative path="AudioResults.txt") -> (appended path=w392:path)
            n189 = Concatenate Strings("Audio Test", w397, w396, w397, w395, w397, w394) -> (w393:string)
            n190 = call "File.Delete File if Exists.vi"("Path"=w392) -> ("error out"=w390:errorcluster, "Path Out"=w391:path)  [unwired: 9 in]
            "Output file" <- w391
            n191 = Write to Text File(file (use dialog)=w391, text=w393, error in=w390) -> (error out=w389:errorcluster)  [unwired: 1 in, 2 out]
          }
          frame "Exit App" {
            n192 = call <vilib>:"Q.Enqueue Exit.vi"("Q In"=w405) -> ()  [unwired: 9 in, 2 out]
          }
        }
      }
      frame "Error", Default {
        n193 = case shown="\"Error\"" w410 {
          tunnel: w409 -> [w412 w414]
          tunnel: w408 -> [_ w415]
          tunnel: [w412 w413] -> w407
          frame Default {
          }
          frame "Error" {
            n194 = Variant To Data(type=w414, Variant=w415) -> (data=w413:errorcluster)  [unwired: 1 in, 1 out]
          }
        }
        "error out" <- w407
      }
      frame "Exit" {
        n195 = Generate User Event(user event=w417, event data cluster=TRUE ("event data")) -> ()  [unwired: 2 in, 2 out]
      }
    }
  }
